vi "Trivial_client.vi"() -> (0 "Difference":dbl format="%.2f", 1 "Server time":dbl format="%.2f")   [LabVIEW 2010]
doc: "This is an example of using features of the VI Server as a client. It shows how you might browse from one or more applications that may be exporting data from one or more data stations. \n\nThe example shows how to query a server for its list of exported VIs, how to get references to the VIs, and how call them with the Call By Reference function."
uses:
  Anemometry/Anemometry Sub Vis/Globals/Preference_global.vi
panel:
  out "Iterations":i32
  out "error Out":errorcluster
  in  "trivial.vi type":refnum<vi>
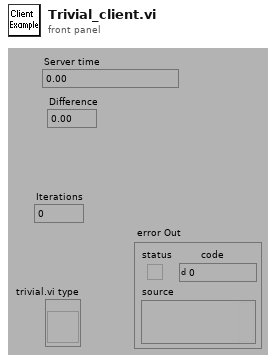
[diagram p1: front panel]
types:
  T1 = typedef "Server_Comms.ctl" = enum16{"Server Link Healthy", "Do Not Link To Server"}
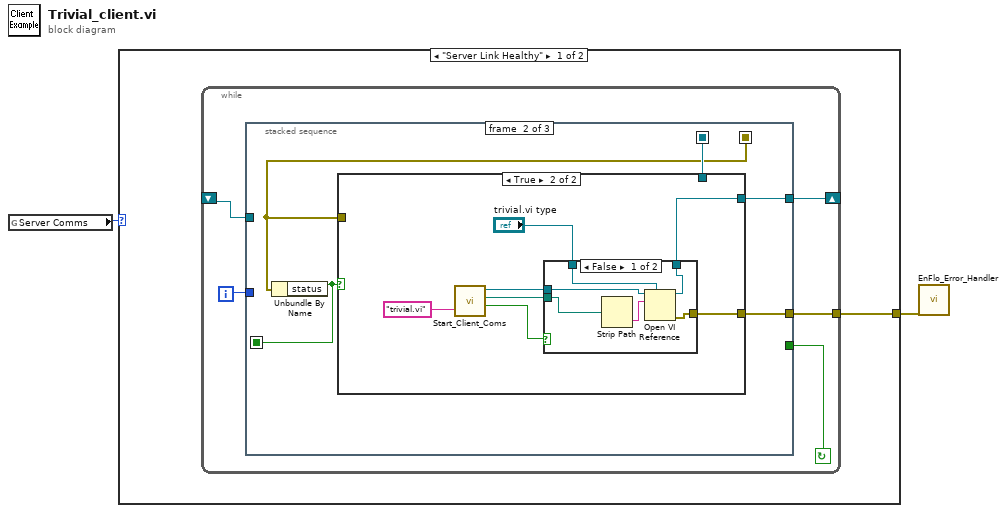
[diagram p0: block diagram]
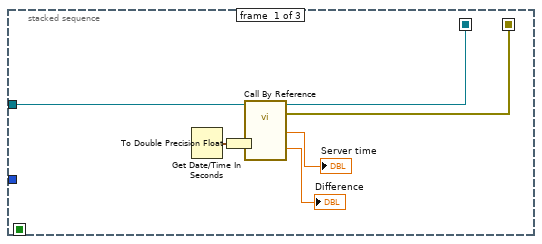
[diagram p2: hidden frame]
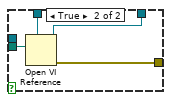
[diagram p4: hidden frame]
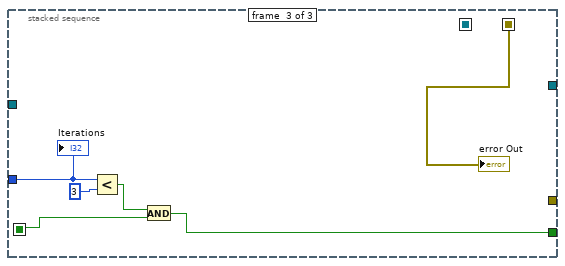
[diagram p5: hidden frame]
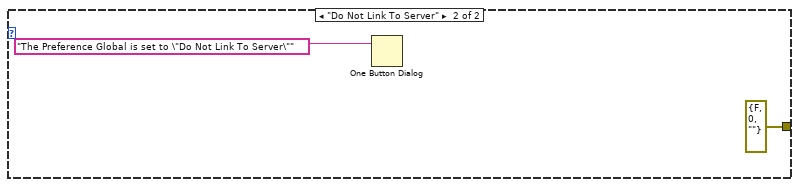
[diagram p6: hidden frame]
diagram:
  n1 = global read "Preference_global.vi" "Server Comms"() -> (w2:T1)
  n2 = case shown="\"Server Link Healthy\"" w2 {
    tunnel: [w3 errorcluster {"status"=FALSE, "code"=0, "source"=""}] -> w1
    frame "Server Link Healthy" {
      n3 = while {
        tunnel: [w4] -> w3
        shift-left: _ -> [w8]
        shift-right: [w7] -> _
        i -> [w6]
        stop <- w5 continue-if-true
        n4 = stacked-sequence {
          seq-local: [w10 _ _] -> [_ w19 _]
          seq-local: [w12 _ _] -> [_ w16 w41]
          seq-local: [_ w18 _] -> [_ _ w42]
          tunnel: w8 -> [w11 _ _]
          tunnel: [_ w20 _] -> w7
          tunnel: w6 -> [_ _ w43]
          tunnel: [_ _ w40] -> w5
          tunnel: [_ w17 _] -> w4
          frame #0 {
            n5 = Get Date/Time In Seconds() -> (seconds since 1Jan1904=w9:timestamp)
            n6 = To Double Precision Float(number=w9) -> (double precision float=w13:dbl)
            n7 = call-by-ref "?"(reference=w11, "Client time"=w13) -> (reference out=w10:refnum<vi>, error out=w12:errorcluster, "Server time"=→"Server time":dbl, "Difference"=→"Difference":dbl)  [unwired: 1 in]
          }
          frame #1 {
            n8 = Unbundle By Name(w16) -> ("status"=w18:bool)
            n9 = case shown="True" w18 {
              tunnel: [w22 w25] -> w20
              tunnel: w19 -> [w22 _]
              tunnel: [w21 w23] -> w17
              tunnel: w16 -> [w21 _]
              frame False {
              }
              frame True {
                n10 = call "Start_Client_Coms.vi"("VI name to run on server"="trivial.vi") -> ("LabVIEW application reference"=w27:refnum<vi>, "Checked VI name"=w24:path, "Local Call"=w26:bool)  [unwired: 1 in, 1 out]
                n11 = case shown="False" w26 {
                  tunnel: [w32 w39] -> w25
                  tunnel: "trivial.vi type" -> [w31 w38]
                  tunnel: w24 -> [w33 w37]
                  tunnel: w27 -> [w30 _]
                  tunnel: [w34 w36] -> w23
                  frame False {
                    n12 = Strip Path(path=w33) -> (name=w35:string)  [unwired: 1 out]
                    n13 = Open VI Reference(type specifier VI Refnum (for type only)=w31, application reference (local)=w30, vi path=w35) -> (vi reference=w32:refnum<vi>, error out=w34:errorcluster)  [unwired: 1 in, 2 out]
                  }
                  frame True {
                    n14 = Open VI Reference(type specifier VI Refnum (for type only)=w38, vi path=w37) -> (vi reference=w39:refnum<vi>, error out=w36:errorcluster)  [unwired: 1 in, 3 out]
                  }
                }
              }
            }
          }
          frame #2 {
            n15 = Less?(x=w43, y=3) -> (x < y?=w45:bool)
            n16 = And(x=w45, y=w42) -> (x .and. y?=w40:bool)
            "Iterations" <- w43
            "error Out" <- w41
          }
        }
      }
    }
    frame "Do Not Link To Server" {
      n17 = One Button Dialog(message="The Preference Global is set to \"Do Not Link To Server\"") -> ()  [unwired: 2 out]
    }
  }
  n18 = call "EnFlo_Error_Handler.vi"("error in (no error)"=w1) -> ()  [unwired: 2 in, 3 out]
